vi "Trace.vi"(7 "Trace Level":T1(ring)=enum."Debug", 8 "error in (no error)":errorcluster, 9 "Command Processor Message":string, 10 "Command Processor Action":string, 11 "Command Processor Actor in":refnum<class "Command Processor Actor.lvclass">) -> (0 "error out":errorcluster, 3 "Command Processor Actor out":refnum<class "Command Processor Actor.lvclass">)   [LabVIEW 2014, in "Robot Actor Framework.lvlib" / "Command Processor Actor.lvlib" / "Command Processor Actor.lvclass"]
uses:
  Command Processor Actor.lvclass
  Trace/Trace Class/Trace.lvclass
  <vilib>/ActorFramework/Actor/Actor.lvclass/Actor.ctl
  Command Processor Actor.lvclass/Command Processor Actor.ctl
  System Actor/System Actor Messages/Record Trace Msg/Record Trace Msg.lvclass/Record Trace Msg.ctl
  <vilib>/ActorFramework/Message Enqueuer/Message Enqueuer.lvclass/Message Enqueuer.ctl
  <vilib>/ActorFramework/Message Enqueuer/Enqueue.vi
  Utilities/Call Stack to String.vi
  <vilib>/ActorFramework/Message Priority Queue/Priority Enqueue.vi
  System Actor/System Actor Messages/Record Trace Msg/Record Trace Msg.lvclass
  Command Actor/Command Actor Class/Command Actor.lvclass
  <vilib>/ActorFramework/Actor/Actor.lvclass
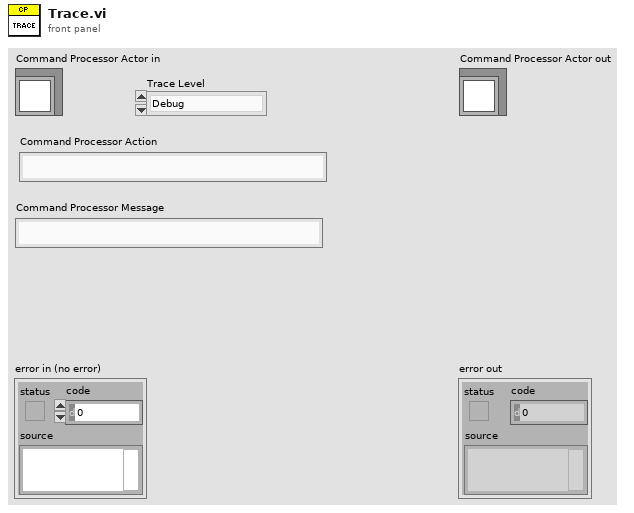
[diagram p1: front panel]
types:
  T1 = enum16{"Critical", "Error", "Warning", "Informational", "Debug"}
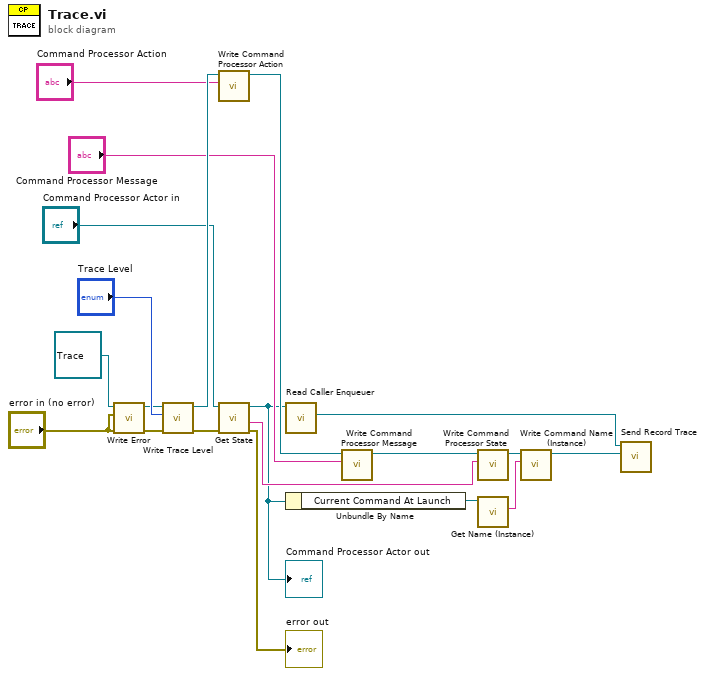
[diagram p0: block diagram]
diagram:
  n1 = call-dynamic "Write Error.vi"("error in (no error)"="error in (no error)", "Error"="error in (no error)", "Trace in"=refnum<class "Trace.lvclass"> refnum ("Robot Actor Framework.lvlib:Trace.lvlib:Trace.lvclass")) -> ("error out"=w3:errorcluster, "Trace out"=w5:refnum<class "Trace.lvclass">)  [unwired: 7 in]
  n2 = call-dynamic "Write Trace Level.vi"("error in (no error)"=w3, "Trace Level"="Trace Level", "Trace in"=w5) -> ("error out"=w2:errorcluster, "Trace out"=w19:refnum<class "Trace.lvclass">)  [unwired: 7 in]
  n3 = call-dynamic "Write Command Processor Action.vi"("Command Processor Action"="Command Processor Action", "Trace in"=w19) -> ("Trace out"=w18:refnum<class "Trace.lvclass">)  [unwired: 8 in, 1 out]
  n4 = call-dynamic "Get State.vi"("error in (no error)"=w2, "Command Processor Actor in"="Command Processor Actor in") -> ("error out"=→"error out":errorcluster, "State String"=w13:string, "Command Processor Actor out"=w12:refnum<class "Command Processor Actor.lvclass">)  [unwired: 7 in]
  "Command Processor Actor out" <- w12
  n5 = call <vilib>:"Read Caller Enqueuer.vi"("Actor"=w12) -> ("Caller Enqueuer"=w20:refnum<class "Message Enqueuer.lvclass">)  [unwired: 10 in]
  n6 = Unbundle By Name(w12) -> ("Current Command At Launch"=w11:refnum<class "Command Actor.lvclass">)
  n7 = call-dynamic "Write Command Processor Message.vi"("Command Processor Message"="Command Processor Message", "Trace in"=w18) -> ("Trace out"=w17:refnum<class "Trace.lvclass">)  [unwired: 8 in, 1 out]
  n8 = call-dynamic "Write Command Processor State.vi"("Command Processor State"=w13, "Trace in"=w17) -> ("Trace out"=w10:refnum<class "Trace.lvclass">)  [unwired: 8 in, 1 out]
  n9 = call-dynamic "Get Name (Instance).vi"("Command Actor in"=w11) -> ("Name (Instance)"=w9:string)  [unwired: 8 in, 2 out]
  n10 = call-dynamic "Write Command Name (Instance).vi"("Command Name (Instance)"=w9, "Trace in"=w10) -> ("Trace out"=w8:refnum<class "Trace.lvclass">)  [unwired: 8 in, 1 out]
  n11 = call "Send Record Trace.vi"("Trace"=w8, "Message Enqueuer"=w20) -> ()  [unwired: 8 in, 2 out]
